vi "NF LI56xx GettingStarted.vi"() -> ()   [LabVIEW 2019]
doc: "This VI provide limited control for LI5645,LI5650,LI5655,LI5660."
uses:
  CTR/Status.ctl
panel:
  out "status":dbl
  out "DATA4":string
  out "DATA3":string
  out "DATA2":string
  out "DATA1":string
  in  "Reference":T1
  in  "VISA resource name":refnum<visa-resource-name>
  in  "Frequency":dbl=1000.0 format="%_7p"
  in  "Time Constant":dbl=1.0 caption="TimeConstantValue" min=1e-06 max=50000.0
  in  "Sensitivity":dbl=1.0 caption="VoltageSensitivity" min=1e-08 max=1.0 step=0.1
  in  "Amp":dbl min=0.0 max=1.0 format="%_4p"
  in  "Range":enum16{"10E-3", "100E-3", "1"}(ring)
  in  "Phase":dbl min=-180.0 max=179.999 step=0.001 format="%.3g"
  in  "Slope":enum16{"6", "12", "18", "24"}(ring)
  in  "Filter":enum16{"EXPonential", "MOVing"}(ring)
  in  "Dynamic Reserve":enum16{"HIGH", "MEDium", "LOW"}(ring)
  in  "DATA4":enum16{"IMAGinary", "PHASe"}(ring)=enum."PHASe"
  in  "DATA3":enum16{"REAL", "MLINear"}(ring)=enum."MLINear"
  in  "DATA2":enum16{"IMAGinary", "PHASe", "AUX1", "AUX2"}(ring)
  in  "DATA1":enum8{"REAL", "MLINear", "NOISe", "AUX1"}(ring)
  in  "SIG":T2
  out "measurement data":dbl[](array[numeric]) format="%#_7p"
  # "LI56xx GettingStarted.vi"
  # "Measurement Data"
  # "Setting"
  # "*"
  # "[Vrms or Arms]"
  # "[Vrms]"
  # "*"
  # "[V]"
  # "[s]"
  # "[degree]"
  # "[Hz]"
  # "[dB/oct]"
  # "*Sensitivity and Time Constant are Rounded to apply to arbitrary values specified at sending message"
  # "[V/A]"
  # "[ohm]"
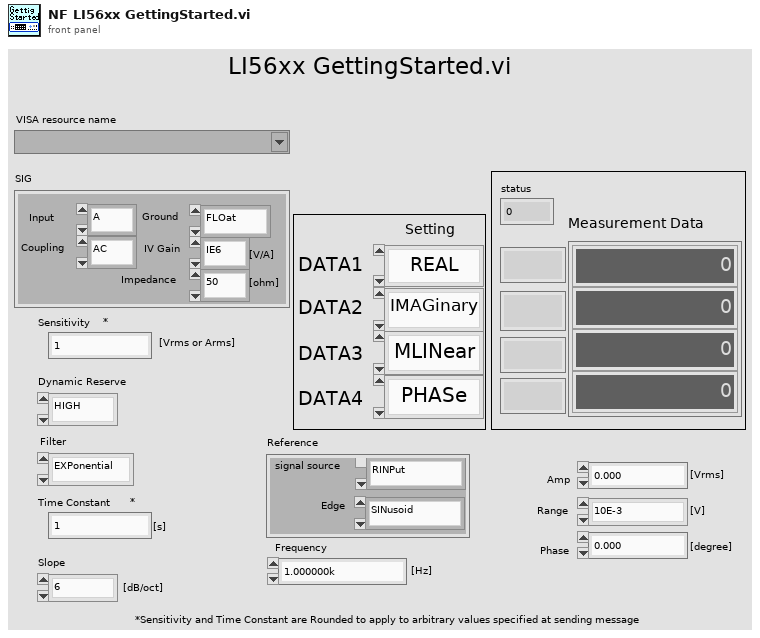
[diagram p1: front panel]
types:
  T1 = cluster{"signal source":enum16{"RINPut", "IOSC", "SINPut"}, "Edge":enum16{"SINusoid", "TPOS", "TNEG"}}
  T2 = cluster{"Input":enum16{"A", "AB", "C", "I", "HF"}, "Coupling":enum16{"AC", "DC"}, "Ground":enum16{"FLOat", "GROund"}, "IV Gain":enum16{"IE6", "IE8"}, "Impedance":enum16{"50", "1E6"}}
  T3 = typedef "Status.ctl" = enum16{"Init", "Data1", "Data2", "Data3", "Data4", "OSC", "Input", "Sense", "DR", "TC", "Filter", "Slope", "Ref", "Freq", "Phase", "Meas", "Stop"}
  T4 = enum16{"REAL", "MLINear", "IMAGinary", "PHASe", "NOISe", "AUX1", "REAL2", "MLINear2"}
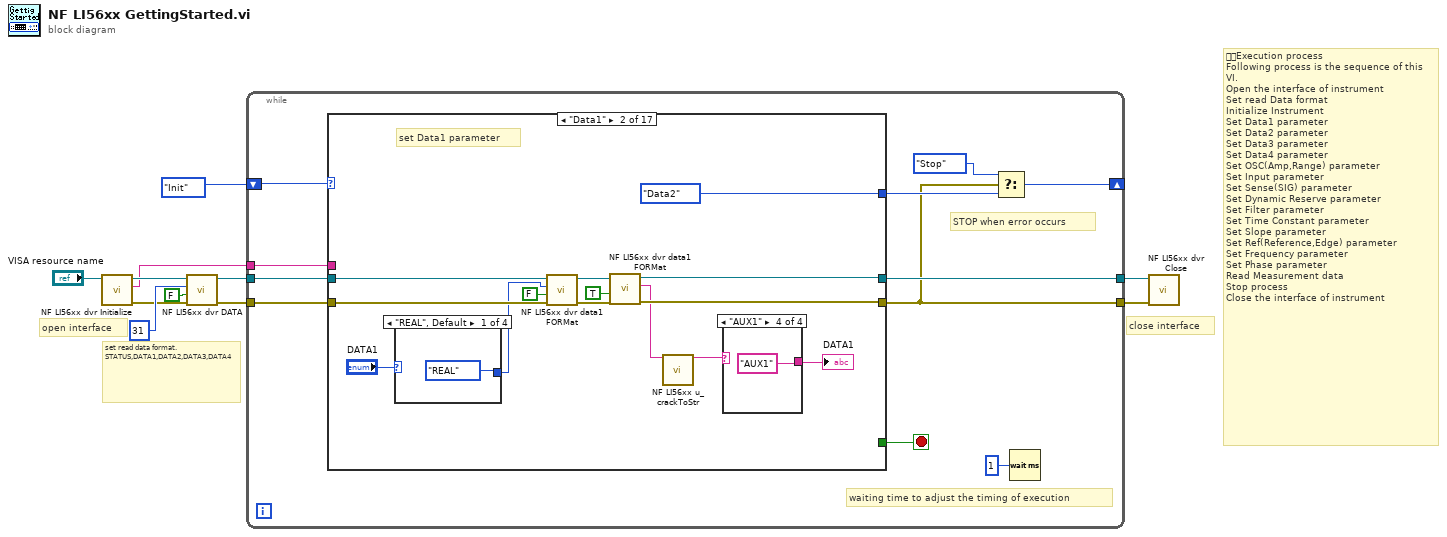
[diagram p0: block diagram]
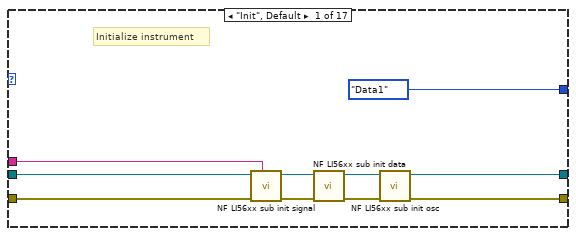
[diagram p2: hidden frame]
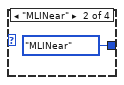
[diagram p3: hidden frame]
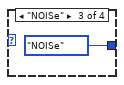
[diagram p4: hidden frame]
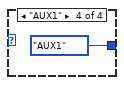
[diagram p5: hidden frame]
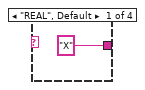
[diagram p6: hidden frame]
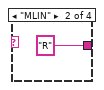
[diagram p7: hidden frame]
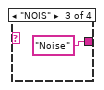
[diagram p8: hidden frame]
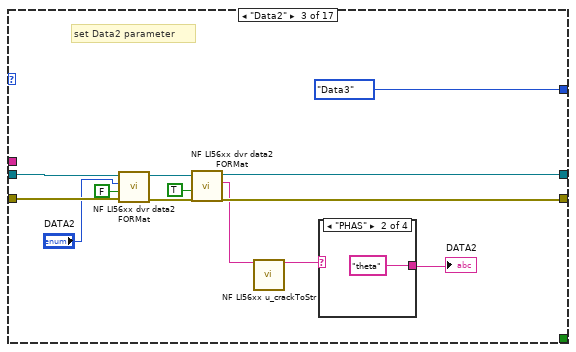
[diagram p9: hidden frame]
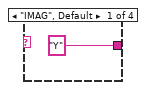
[diagram p10: hidden frame]
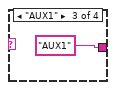
[diagram p11: hidden frame]
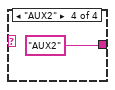
[diagram p12: hidden frame]
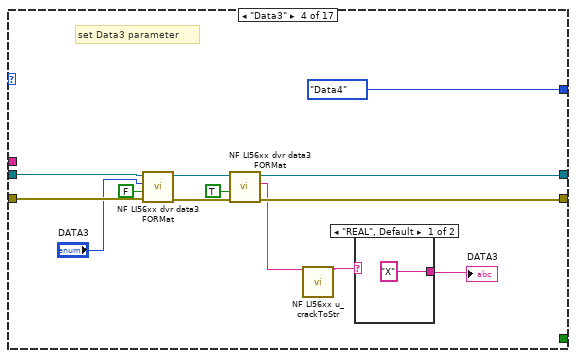
[diagram p13: hidden frame]
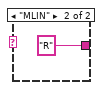
[diagram p14: hidden frame]
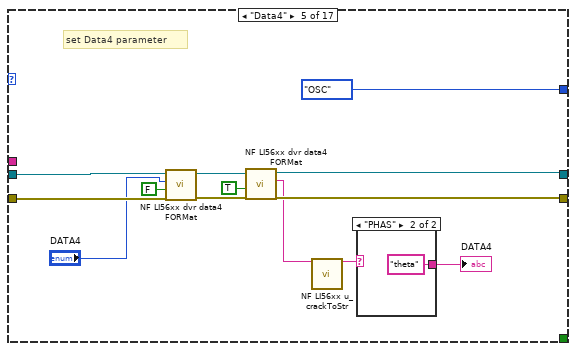
[diagram p15: hidden frame]
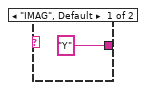
[diagram p16: hidden frame]
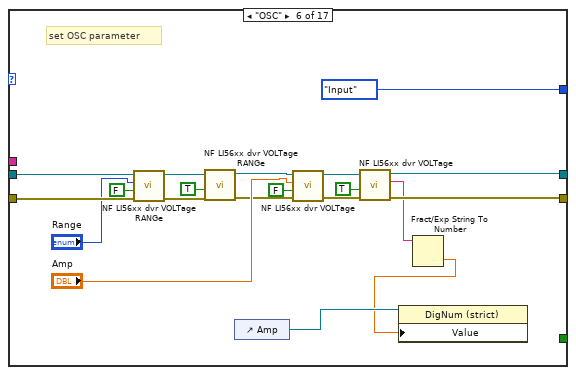
[diagram p17: hidden frame]
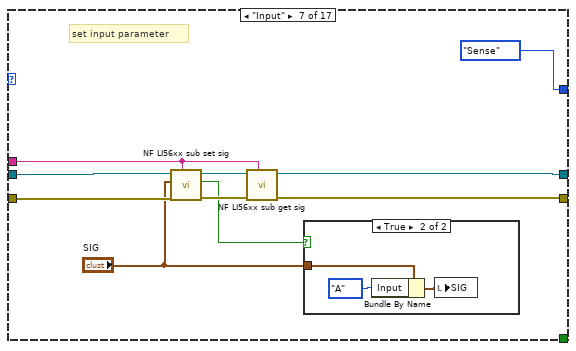
[diagram p18: hidden frame]
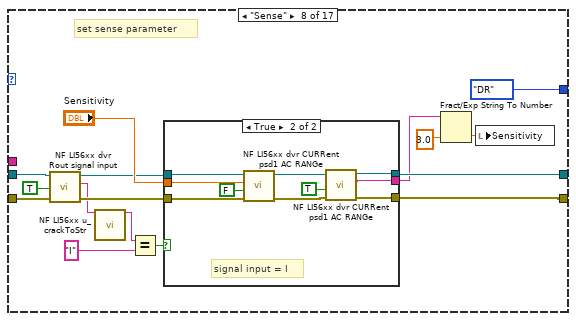
[diagram p20: hidden frame]
diagram:
  # "Execution process\nFollowing process is the sequence of this VI.\nOpen the interface of instrument\nSet read Data format\nInitialize Instrument\nSet Data1 parameter\nSet Data2 parameter\nSet Data3 parameter\nSet Data4 parameter\nSet OSC(Amp,Range) parameter\nSet Input parameter\nSet Sense(SIG) parameter\nSet Dynamic Reserve parameter\nSet Filter parameter\nSet Time Constant parameter\nSet Slope parameter\nSet Ref(Reference,Edge) parameter\nSet Frequency parameter\nSet Phase parameter\nRead Measurement data\nStop process\nClose the interface of instrument"
  # "close interface"
  # "open interface"
  # "set read data format.\nSTATUS,DATA1,DATA2,DATA3,DATA4"
  n1 = call "NF LI56xx dvr Initialize.vi"("VISA resource name"="VISA resource name") -> ("error out"=w9:errorcluster, "type"=w1:string, "VISA resource name out"=w7:refnum<visa-resource-name>)  [unwired: 8 in]
  n2 = call "NF LI56xx dvr DATA.vi"("error in"=w9, "Read(F)"=FALSE, "set measurement data"=31 ("DataReadoutType"), "VISA resource name"=w7) -> ("error out"=w8:errorcluster, "VISA resource name copy"=w5:refnum<visa-resource-name>)  [unwired: 5 in, 1 out]
  n3 = while {
    tunnel: w8 -> [w22]
    tunnel: [w21] -> w3
    tunnel: [w15] -> w4
    shift-right: [w17] -> _
    shift-left: Status."Init" ("Status") -> [w19]
    tunnel: w5 -> [w13]
    tunnel: w1 -> [w12]
    stop <- w20 stop-if-true
    # "STOP when error occurs"
    # "waiting time to adjust the timing of execution"
    n4 = case shown="\"Data1\"" w19 {
      tunnel: w22 -> [w27 w45 w66 w83 w98 w116 w131 w144 w179 w191 w201 w212 w230 w244 w254 w261 w283]
      tunnel: [w25 w38 w58 w75 w91 w102 w126 w147 w171 w184 w194 w204 w220 w234 w247 w276 w281] -> w21
      tunnel: [w26 w39 w64 w81 w96 w111 w127 w146 w173 w185 w195 w207 w222 w235 w252 w275 w282] -> w15
      tunnel: [_ _ _ _ _ _ _ _ _ _ _ _ _ _ _ _ TRUE] -> w20
      tunnel: [Status."Data1" ("Status") Status."Data2" ("Status") Status."Data3" ("Status") Status."Data4" ("Status") Status."OSC" ("Status") Status."Input" ("Status") Status."Sense" ("Status") Status."DR" ("Status") Status."Filter" ("Status") Status."Slope" ("Status") Status."TC" ("Status") Status."Ref" ("Status") w217 Status."Phase" ("Status") Status."Meas" ("Status") Status."Stop" ("Status") Status."Init" ("Status")] -> w16
      tunnel: w13 -> [w24 w44 w62 w77 w95 w114 w130 w143 w178 w192 w202 w211 w231 w245 w255 w262 w281]
      tunnel: w12 -> [w23 _ _ _ _ _ w125 _ _ _ _ _ _ _ _ _ _]
      frame "Init", Default {
        # "Initialize instrument"
        n5 = call "NF LI56xx sub init signal.vi"("Type"=w23, "error in"=w27, "VISA resource name"=w24) -> ("error out"=w29:errorcluster, "VISA resource name copy"=w31:refnum<visa-resource-name>)  [unwired: 7 in]
        n6 = call "NF LI56xx sub init data.vi"("error in"=w29, "VISA resource name"=w31) -> ("error out"=w28:errorcluster, "VISA resource name copy"=w30:refnum<visa-resource-name>)  [unwired: 8 in]
        n7 = call "NF LI56xx sub init osc.vi"("error in"=w28, "VISA resource name"=w30) -> ("error out"=w26:errorcluster, "VISA resource name copy"=w25:refnum<visa-resource-name>)  [unwired: 8 in]
      }
      frame "Data1" {
        # "set Data1 parameter"
        n8 = case shown="\"REAL\", Default" "DATA1" {
          tunnel: [T4."REAL" T4."MLINear" T4."NOISe" T4."AUX1"] -> w33
          frame "REAL", Default {
          }
          frame "MLINear" {
          }
          frame "NOISe" {
          }
          frame "AUX1" {
          }
        }
        n9 = call "NF LI56xx dvr data1 FORMat.vi"("error in"=w45, "Read(F)"=FALSE, "set measurement \nparameters format"=w33, "VISA resource name"=w44) -> ("error out"=w42:errorcluster, "VISA resource name copy"=w41:refnum<visa-resource-name>)  [unwired: 5 in, 1 out]
        n10 = call "NF LI56xx dvr data1 FORMat.vi"("error in"=w42, "Read(F)"=TRUE, "VISA resource name"=w41) -> ("error out"=w39:errorcluster, "query measurement \nparameters format"=w35:string, "VISA resource name copy"=w38:refnum<visa-resource-name>)  [unwired: 6 in]
        n11 = call "NF LI56xx u_crackToStr.vi"("input string"=w35) -> ("output string"=w36:string)  [unwired: 18 in]
        n12 = case shown="\"AUX1\"" w36 {
          tunnel: ["X" "R" "Noise" "AUX1"] -> w37
          frame "REAL", Default {
          }
          frame "MLIN" {
          }
          frame "NOIS" {
          }
          frame "AUX1" {
          }
        }
        "DATA1" <- w37
      }
      frame "Data2" {
        # "set Data2 parameter"
        n13 = call "NF LI56xx dvr data2 FORMat.vi"("error in"=w66, "Read(F)"=FALSE, "set measurement \nparameters format"="DATA2", "VISA resource name"=w62) -> ("error out"=w65:errorcluster, "VISA resource name copy"=w63:refnum<visa-resource-name>)  [unwired: 5 in, 1 out]
        n14 = call "NF LI56xx dvr data2 FORMat.vi"("error in"=w65, "Read(F)"=TRUE, "VISA resource name"=w63) -> ("error out"=w64:errorcluster, "query measurement\nparameters format"=w55:string, "VISA resource name copy"=w58:refnum<visa-resource-name>)  [unwired: 6 in]
        n15 = call "NF LI56xx u_crackToStr.vi"("input string"=w55) -> ("output string"=w56:string)  [unwired: 18 in]
        n16 = case shown="\"PHAS\"" w56 {
          tunnel: ["Y" "theta" "AUX1" "AUX2"] -> w57
          frame "IMAG", Default {
          }
          frame "PHAS" {
          }
          frame "AUX1" {
          }
          frame "AUX2" {
          }
        }
        "DATA2" <- w57
      }
      frame "Data3" {
        # "set Data3 parameter"
        n17 = call "NF LI56xx dvr data3 FORMat.vi"("error in"=w83, "Read(F)"=FALSE, "set measurement \nparameters format"="DATA3", "VISA resource name"=w77) -> ("error out"=w82:errorcluster, "VISA resource name copy"=w76:refnum<visa-resource-name>)  [unwired: 5 in, 1 out]
        n18 = call "NF LI56xx dvr data3 FORMat.vi"("error in"=w82, "Read(F)"=TRUE, "VISA resource name"=w76) -> ("error out"=w81:errorcluster, "query measurement \nparameters format"=w73:string, "VISA resource name copy"=w75:refnum<visa-resource-name>)  [unwired: 6 in]
        n19 = call "NF LI56xx u_crackToStr.vi"("input string"=w73) -> ("output string"=w72:string)  [unwired: 18 in]
        n20 = case shown="\"REAL\", Default" w72 {
          tunnel: ["X" "R"] -> w74
          frame "REAL", Default {
          }
          frame "MLIN" {
          }
        }
        "DATA3" <- w74
      }
      frame "Data4" {
        # "set Data4 parameter"
        n21 = call "NF LI56xx dvr data4 FORMat.vi"("error in"=w98, "Read(F)"=FALSE, "set measurement \nparameters format"="DATA4", "VISA resource name"=w95) -> ("error out"=w97:errorcluster, "VISA resource name copy"=w92:refnum<visa-resource-name>)  [unwired: 5 in, 1 out]
        n22 = call "NF LI56xx dvr data4 FORMat.vi"("error in"=w97, "Read(F)"=TRUE, "VISA resource name"=w92) -> ("error out"=w96:errorcluster, "query measurement \nparameters format"=w88:string, "VISA resource name copy"=w91:refnum<visa-resource-name>)  [unwired: 6 in]
        n23 = call "NF LI56xx u_crackToStr.vi"("input string"=w88) -> ("output string"=w87:string)  [unwired: 18 in]
        n24 = case shown="\"PHAS\"" w87 {
          tunnel: ["Y" "theta"] -> w89
          frame "IMAG", Default {
          }
          frame "PHAS" {
          }
        }
        "DATA4" <- w89
      }
      frame "OSC" {
        # "set OSC parameter"
        n25 = call "NF LI56xx dvr VOLTage RANGe.vi"("error in"=w116, "Read(F)"=FALSE, "set AC Voltage"="Range", "VISA resource name"=w114) -> ("error out"=w112:errorcluster, "VISA resource name copy"=w113:refnum<visa-resource-name>)  [unwired: 5 in, 1 out]
        n26 = call "NF LI56xx dvr VOLTage RANGe.vi"("error in"=w112, "Read(F)"=TRUE, "VISA resource name"=w113) -> ("error out"=w109:errorcluster, "VISA resource name copy"=w108:refnum<visa-resource-name>)  [unwired: 6 in, 1 out]
        n27 = control-ref of="Amp"() -> (w120:refnum<vi>)
        n28 = call "NF LI56xx dvr VOLTage.vi"("error in"=w109, "Read(F)"=FALSE, "set AC Voltage"="Amp", "VISA resource name"=w108) -> ("error out"=w110:errorcluster, "VISA resource name copy"=w107:refnum<visa-resource-name>)  [unwired: 5 in, 1 out]
        n29 = call "NF LI56xx dvr VOLTage.vi"("error in"=w110, "Read(F)"=TRUE, "VISA resource name"=w107) -> ("error out"=w111:errorcluster, "query AC Voltage"=w104:string, "VISA resource name copy"=w102:refnum<visa-resource-name>)  [unwired: 6 in]
        n30 = Fract/Exp String To Number(string=w104) -> (number=w103:dbl)  [unwired: 3 in, 1 out]
        n31 = property class="DigNum (strict)"(reference=w120, "Value"=w103) -> ()  [unwired: 1 in, 2 out]
      }
      frame "Input" {
        # "set input parameter"
        n32 = call "NF LI56xx sub set sig.vi"("Type"=w125, "error in"=w131, "Input"="SIG", "VISA resource name"=w130) -> ("error out"=w128:errorcluster, "change input type"=w122:bool, "VISA resource name copy"=w129:refnum<visa-resource-name>)  [unwired: 5 in]
        n33 = call "NF LI56xx sub get sig.vi"("Type"=w125, "error in"=w128, "VISA resource name"=w129) -> ("error out"=w127:errorcluster, "VISA resource name copy"=w126:refnum<visa-resource-name>)  [unwired: 6 in, 1 out]
        n34 = case shown="True" w122 {
          tunnel: "SIG" -> [_ w134]
          frame False {
          }
          frame True {
            n35 = Bundle By Name(cluster=w134, "Input"=enum16{"A", "AB", "C", "I", "HF"}."A") -> (w133:T2)
            n36 = local write "SIG"(w133) -> ()
          }
        }
      }
      frame "Sense" {
        # "set sense parameter"
        n37 = call "NF LI56xx dvr Rout signal input.vi"("error in"=w144, "Read(F)"=TRUE, "VISA resource name"=w143) -> ("error out"=w142:errorcluster, "query signal input"=w135:string, "VISA resource name copy"=w141:refnum<visa-resource-name>)  [unwired: 6 in]
        n38 = call "NF LI56xx u_crackToStr.vi"("input string"=w135) -> ("output string"=w136:string)  [unwired: 18 in]
        n39 = Equal?(x=w136, y="I") -> (x = y?=w149:bool)
        n40 = case shown="True" w149 {
          tunnel: w141 -> [w160 w167]
          tunnel: w142 -> [w158 w168]
          tunnel: [w154 w165] -> w147
          tunnel: [w156 w169] -> w146
          tunnel: "Sensitivity" -> [w159 w163]
          tunnel: [w155 w164] -> w140
          frame False {
            # "signal input = A,AB,C"
            n41 = call "NF LI56xx dvr VOLTage psd1 AC RANGe.vi"("error in"=w158, "Read(F)"=FALSE, "set sensitivity"=w159, "VISA resource name"=w160) -> ("error out"=w157:errorcluster, "VISA resource name copy"=w153:refnum<visa-resource-name>)  [unwired: 5 in, 1 out]
            n42 = call "NF LI56xx dvr VOLTage psd1 AC RANGe.vi"("error in"=w157, "Read(F)"=TRUE, "VISA resource name"=w153) -> ("error out"=w156:errorcluster, "query sensitivity"=w155:string, "VISA resource name copy"=w154:refnum<visa-resource-name>)  [unwired: 6 in]
          }
          frame True {
            # "signal input = I"
            n43 = call "NF LI56xx dvr CURRent psd1 AC RANGe.vi"("error in"=w168, "Read(F)"=FALSE, "set sensitivity"=w163, "VISA resource name"=w167) -> ("error out"=w170:errorcluster, "VISA resource name copy"=w166:refnum<visa-resource-name>)  [unwired: 5 in, 1 out]
            n44 = call "NF LI56xx dvr CURRent psd1 AC RANGe.vi"("error in"=w170, "Read(F)"=TRUE, "VISA resource name"=w166) -> ("error out"=w169:errorcluster, "query sensitivity"=w164:string, "VISA resource name copy"=w165:refnum<visa-resource-name>)  [unwired: 6 in]
          }
        }
        n45 = Fract/Exp String To Number(string=w140, default (0 dbl)=3.0 ("デフォルト （0 DBL）")) -> (number=w138:dbl)  [unwired: 2 in, 1 out]
        n46 = local write "Sensitivity"(w138) -> ()
      }
      frame "DR" {
        # "set dynamic reserve parameter"
        n47 = call "NF LI56xx dvr DREServe.vi"("error in"=w179, "Read(F)"=FALSE, "set dynamic reserve"="Dynamic Reserve", "VISA resource name"=w178) -> ("error out"=w176:errorcluster, "VISA resource name copy"=w177:refnum<visa-resource-name>)  [unwired: 5 in, 1 out]
        n48 = call "NF LI56xx dvr DREServe.vi"("error in"=w176, "Read(F)"=TRUE, "VISA resource name"=w177) -> ("error out"=w173:errorcluster, "VISA resource name copy"=w171:refnum<visa-resource-name>)  [unwired: 6 in, 1 out]
      }
      frame "TC" {
        # "set time constant parameter"
        n49 = call "NF LI56xx dvr FILTer psd1 TCONstant.vi"("error in"=w191, "Read(F)"=FALSE, "set time constant"="Time Constant", "VISA resource name"=w192) -> ("error out"=w187:errorcluster, "VISA resource name copy"=w188:refnum<visa-resource-name>)  [unwired: 5 in, 1 out]
        n50 = call "NF LI56xx dvr FILTer psd1 TCONstant.vi"("error in"=w187, "Read(F)"=TRUE, "VISA resource name"=w188) -> ("error out"=w185:errorcluster, "query time constnat"=w181:string, "VISA resource name copy"=w184:refnum<visa-resource-name>)  [unwired: 6 in]
        n51 = Fract/Exp String To Number(string=w181, default (0 dbl)=3.0 ("デフォルト （0 DBL）")) -> (number=w182:dbl)  [unwired: 2 in, 1 out]
        n52 = local write "Time Constant"(w182) -> ()
      }
      frame "Filter" {
        # "set filter parameter"
        n53 = call "NF LI56xx dvr FILTer psd1 TYPE.vi"("error in"=w201, "Read(F)"=FALSE, "set filter slope"="Filter", "VISA resource name"=w202) -> ("error out"=w198:errorcluster, "VISA resource name copy"=w199:refnum<visa-resource-name>)  [unwired: 5 in, 1 out]
        n54 = call "NF LI56xx dvr FILTer psd1 TYPE.vi"("error in"=w198, "Read(F)"=TRUE, "VISA resource name"=w199) -> ("error out"=w195:errorcluster, "VISA resource name copy"=w194:refnum<visa-resource-name>)  [unwired: 6 in, 1 out]
      }
      frame "Slope" {
        # "set slope parameter"
        n55 = call "NF LI56xx dvr FILTer psd1 SLOPe.vi"("error in"=w212, "Read(F)"=FALSE, "set filter slope"="Slope", "VISA resource name"=w211) -> ("error out"=w206:errorcluster, "VISA resource name copy"=w208:refnum<visa-resource-name>)  [unwired: 5 in, 1 out]
        n56 = call "NF LI56xx dvr FILTer psd1 SLOPe.vi"("error in"=w206, "Read(F)"=TRUE, "VISA resource name"=w208) -> ("error out"=w207:errorcluster, "VISA resource name copy"=w204:refnum<visa-resource-name>)  [unwired: 6 in, 1 out]
      }
      frame "Ref" {
        w221 = TRUE ("Read(F)")
        w227 = FALSE ("Read(F)")
        # "ser reference parameter"
        n57 = Unbundle By Name("Reference") -> ("signal source"=w215:enum16{"RINPut", "IOSC", "SINPut"}, "Edge"=w218:enum16{"SINusoid", "TPOS", "TNEG"})
        n58 = call "NF LI56xx dvr Rout2.vi"("error in"=w230, "Read(F)"=w227, "set reference signal \nsource"=w215, "VISA resource name"=w231) -> ("error out"=w228:errorcluster, "VISA resource name copy"=w229:refnum<visa-resource-name>)  [unwired: 5 in, 1 out]
        n59 = call "NF LI56xx dvr INPut2 TYPE.vi"("error in"=w228, "Read(F)"=w227, "set reference signal\nwaveform"=w218, "VISA resource name"=w229) -> ("error out"=w224:errorcluster, "VISA resource name copy"=w226:refnum<visa-resource-name>)  [unwired: 5 in, 1 out]
        n60 = Equal?(x=0, y=w215) -> (x = y?=w216:bool)
        n61 = call "NF LI56xx dvr Rout2.vi"("error in"=w224, "Read(F)"=w221, "VISA resource name"=w226) -> ("error out"=w223:errorcluster, "VISA resource name copy"=w225:refnum<visa-resource-name>)  [unwired: 6 in, 1 out]
        n62 = case shown="True" w216 {
          tunnel: [Status."Freq" ("Status") Status."Phase" ("Status")] -> w217
          frame False {
          }
          frame True {
          }
        }
        n63 = call "NF LI56xx dvr INPut2 TYPE.vi"("error in"=w223, "Read(F)"=w221, "VISA resource name"=w225) -> ("error out"=w222:errorcluster, "VISA resource name copy"=w220:refnum<visa-resource-name>)  [unwired: 6 in, 1 out]
      }
      frame "Freq" {
        w242 = FALSE ("Read(F)")
        # "this VI disable harmonic measurement function"
        # "set frequency parameter"
        n64 = call "NF LI56xx dvr FREQuency psd1.vi"("error in"=w244, "Read(F)"=w242, "set Frequency"="Frequency", "VISA resource name"=w245) -> ("error out"=w243:errorcluster, "VISA resource name copy"=w240:refnum<visa-resource-name>)  [unwired: 5 in, 1 out]
        n65 = call "NF LI56xx dvr FREQuency psd1 HARMonics.vi"("error in"=w243, "Read(F)"=w242, "set harmonic\nmeasuremet"=FALSE ("set harmonic\nmeasuremet"), "VISA resource name"=w240) -> ("error out"=w237:errorcluster, "VISA resource name copy"=w238:refnum<visa-resource-name>)  [unwired: 5 in, 1 out]
        n66 = call "NF LI56xx dvr FREQuency psd1.vi"("error in"=w237, "Read(F)"=TRUE, "VISA resource name"=w238) -> ("error out"=w235:errorcluster, "VISA resource name copy"=w234:refnum<visa-resource-name>)  [unwired: 6 in, 1 out]
      }
      frame "Phase" {
        # "set phase parameter"
        n67 = call "NF LI56xx dvr PHASe psd1.vi"("error in"=w254, "Read(F)"=FALSE, "set phase shift"="Phase", "VISA resource name"=w255) -> ("error out"=w253:errorcluster, "VISA resource name copy"=w251:refnum<visa-resource-name>)  [unwired: 5 in, 1 out]
        n68 = call "NF LI56xx dvr PHASe psd1.vi"("error in"=w253, "Read(F)"=TRUE, "VISA resource name"=w251) -> ("error out"=w252:errorcluster, "VISA resource name copy"=w247:refnum<visa-resource-name>)  [unwired: 6 in, 1 out]
      }
      frame "Meas" {
        # "read measurement data"
        n69 = call "NF LI56xx dvr FORMat.vi"("error in"=w261, "Read(F)"=FALSE, "set data transfer format"=enum16{"ASCii", "REAL", "INTeger"}."ASCii", "VISA resource name"=w262) -> ("error out"=w260:errorcluster, "VISA resource name copy"=w259:refnum<visa-resource-name>)  [unwired: 5 in, 1 out]
        n70 = call "NF LI56xx dvr FORMat.vi"("error in"=w260, "Read(F)"=TRUE, "VISA resource name"=w259) -> ("error out"=w268:errorcluster, "query data transfer format"=w263:string, "VISA resource name copy"=w267:refnum<visa-resource-name>)  [unwired: 6 in]
        n71 = call "NF LI56xx u_crackToStr.vi"("input string"=w263) -> ("output string"=w264:string)  [unwired: 18 in]
        n72 = case shown="\"ASC\", Default" w264 {
          tunnel: [enum16{"ASCii", "REAL", "INTeger"}."ASCii" enum16{"ASCii", "REAL", "INTeger"}."REAL" enum16{"ASCii", "REAL", "INTeger"}."INTeger"] -> w265
          frame "ASC", Default {
          }
          frame "REAL" {
          }
          frame "INT" {
          }
        }
        n73 = call "NF LI56xx dvr qFETCh.vi"("error in"=w268, "VISA resource name"=w267) -> ("error out"=w275:errorcluster, "measurement data"=w272:string, "VISA resource name copy"=w276:refnum<visa-resource-name>)  [unwired: 7 in]
        n74 = call "NF LI56xx u_switch by data type.vi"("Num"=u8 5 ("l"), "data format"=w265, "input string"=w272) -> ("query measurement data"=w271:dbl[])  [unwired: 16 in]
        n75 = Delete From Array(array=w271, index=0 ("Žw•W")) -> (deleted portion=→"status":dbl, array with subset deleted=→"measurement data":dbl[])  [unwired: 1 in]
      }
      frame "Stop" {
        # "stop process"
        n76 = call <vilib>:"Simple Error Handler.vi"("error in (no error)"=w283) -> ("error out"=w282:errorcluster)  [unwired: 4 in, 4 out]
      }
    }
    n77 = Select(t=Status."Stop" ("Status"), s=w15, f=w16) -> (s? t:f=w17:T3)
    n78 = Wait (ms)(milliseconds to wait=u32 1 ("ミリ秒倍数")) -> ()  [unwired: 1 out]
  }
  n79 = call "NF LI56xx dvr Close.vi"("error in (no error)"=w4, "VISA resource name"=w3) -> ()  [unwired: 8 in, 2 out]
